vi "Global_Var_Other.vi"() -> ()   [LabVIEW 2016]
panel:
  in  "Shooter_Limit":dbl
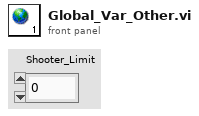
[diagram p1: front panel]
diagram:
